vi "Controller - NStream Read Perform Status.vi"(8 "error in (no error)":errorcluster, 9 "Total Elements":u64, 10 "Available Elmnts":i32, 11 "Status in":string) -> (0 "error out":errorcluster, 3 "Status out":string)   [LabVIEW 2017]
doc: "Perform Entire Status string for logging"
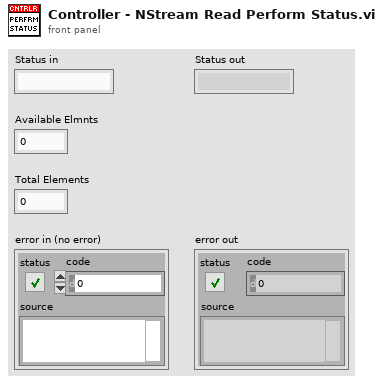
[diagram p1: front panel]
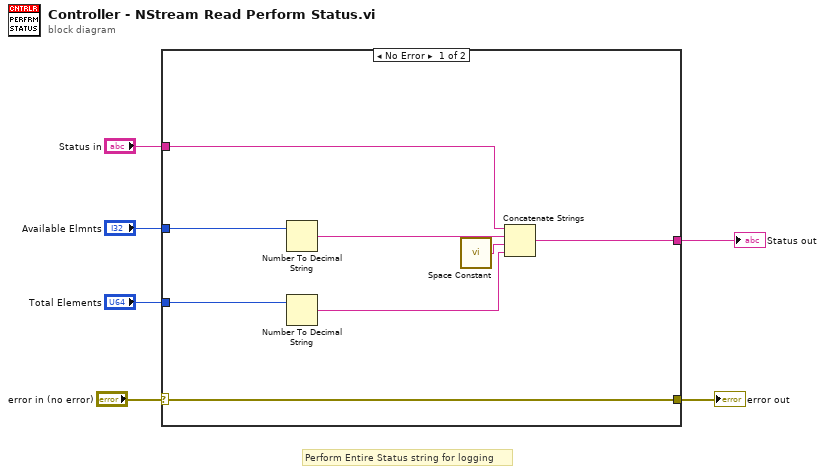
[diagram p0: block diagram]
diagram:
  # "Perform Entire Status string for logging"
  n1 = case shown="No Error" "error in (no error)" {
    selector: "error in (no error)" -> [w14 w16]
    tunnel: [w14 w16] -> w5
    tunnel: "Status in" -> [w10 w15]
    tunnel: "Available Elmnts" -> [w9 _]
    tunnel: "Total Elements" -> [w8 _]
    tunnel: [w7 w15] -> w1
    frame No Error {
      n2 = Number To Decimal String(number=w9) -> (decimal integer string=w13:string)  [unwired: 1 in]
      n3 = Number To Decimal String(number=w8) -> (decimal integer string=w11:string)  [unwired: 1 in]
      n4 = call <vilib>:"Space Constant.vi"() -> ("String"=w12:string)
      n5 = Concatenate Strings(w10, w13, w12, w11) -> (w7:string)
    }
    frame Error {
    }
  }
  "error out" <- w5
  "Status out" <- w1
